vi "GetDBC_CANID.vi"(11 "String":string) -> (3 "字符串":string)   [LabVIEW 2015]
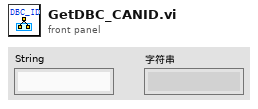
[diagram p1: front panel]
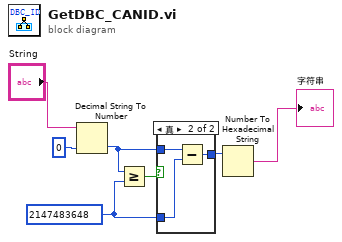
[diagram p0: block diagram]
diagram:
  w6 = u32 2147483648 ("y")
  n1 = Decimal String To Number(string="String", default (0L)=u32 0 ("默认(0 I32)")) -> (number=w5:u32)  [unwired: 1 in, 1 out]
  n2 = Greater Or Equal?(x=w5, y=w6) -> (x >= y?=w7:bool)
  n3 = case shown="真" w7 {
    tunnel: [w8 w11] -> w3
    tunnel: w5 -> [w8 w10]
    tunnel: w6 -> [_ w9]
    frame False {
    }
    frame True {
      n4 = Subtract(x=w10, y=w9) -> (x-y=w11:u32)
    }
  }
  n5 = Number To Hexadecimal String(2:w3) -> (0:→"字符串":string)  [unwired: 1 in]
